vi "Peak_removal_diag.vi"(10 "tolerance (Deviation)":dbl, 11 "Offset removed":cluster{"xi used":dbl[], "yi":dbl[]}(graph)) -> (2 "Tolerance Level":dbl, 3 "XY Graph":cluster{"xi used":dbl[], "yi":dbl[]}(graph))   [LabVIEW 2015]
uses:
  <vilib>/Analysis/NI_AALBase.lvlib
panel:
  out "yi":dbl[](array[numeric])
  out "xi used":dbl[](array[numeric])
  out "XY Graph 2":cluster{"xi used":dbl[], "yi":dbl[]}(graph)
  out "standard deviation":dbl format="%0.2f"
  out "mean":dbl format="%0.2f"
  out "yi 2":dbl[](array[numeric])
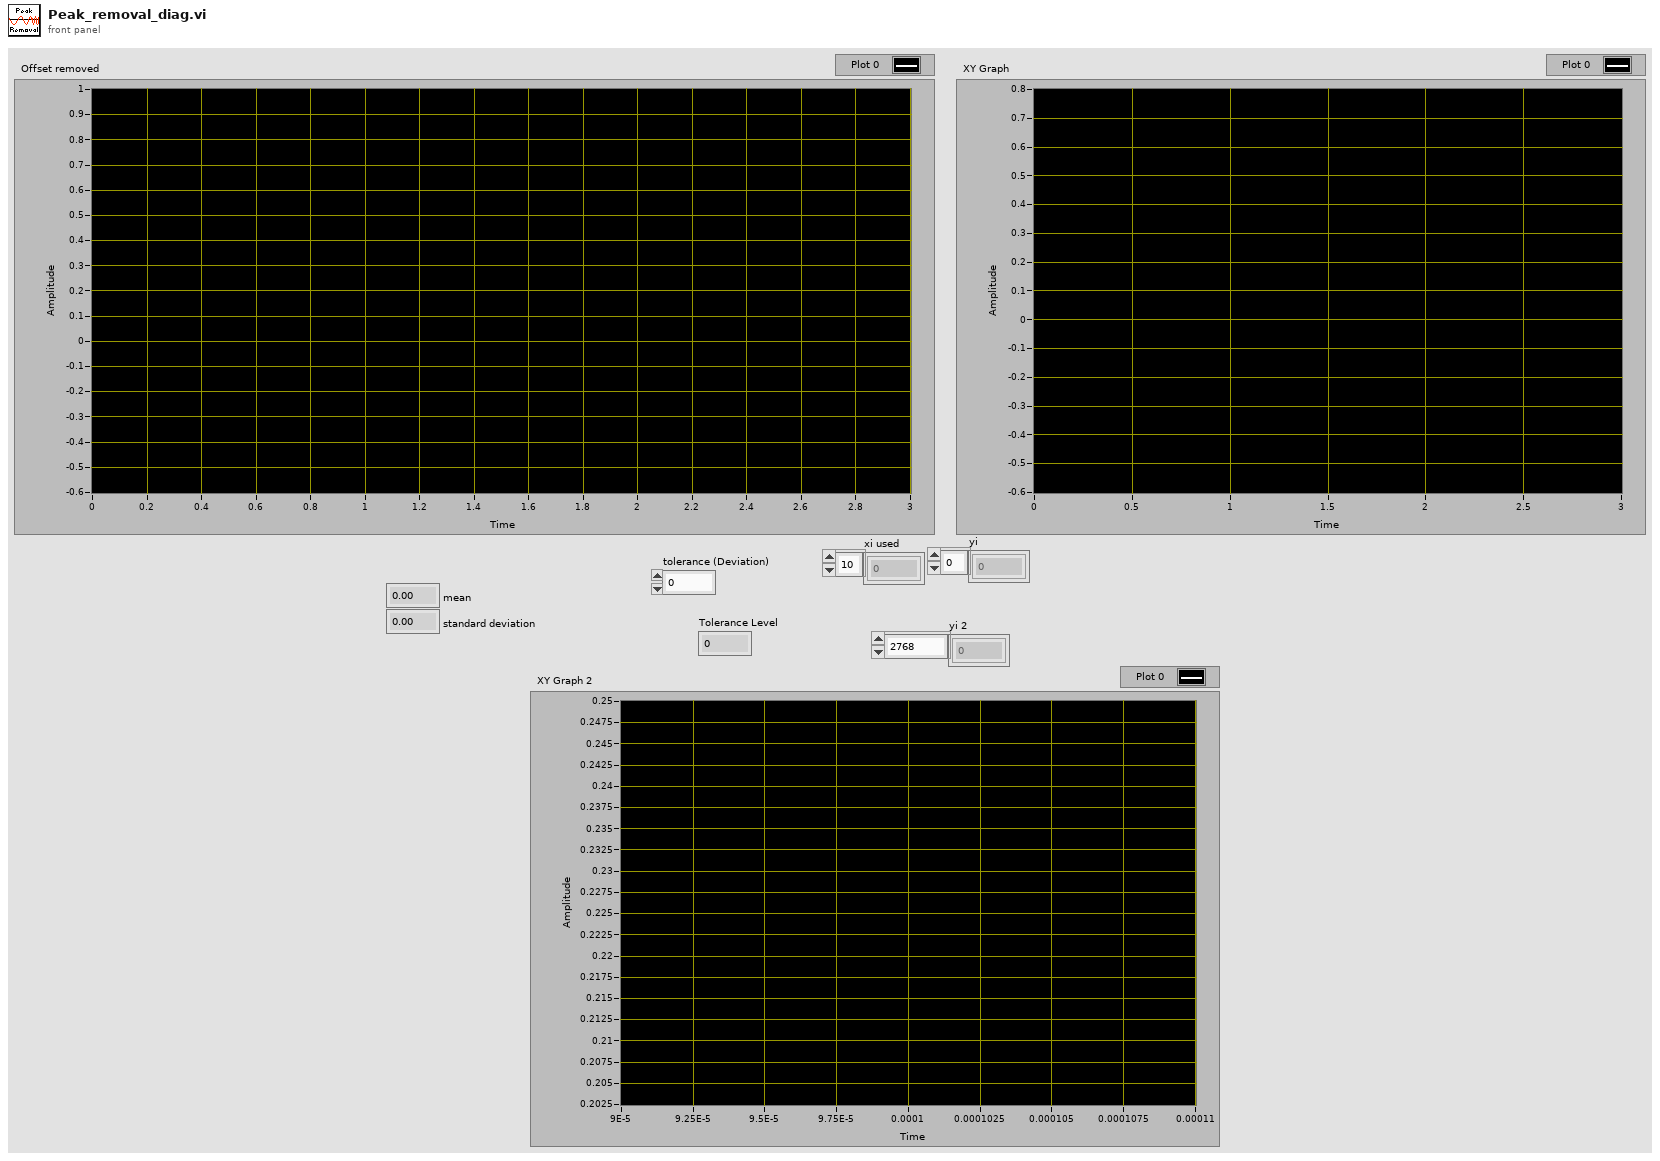
[diagram p1: front panel]
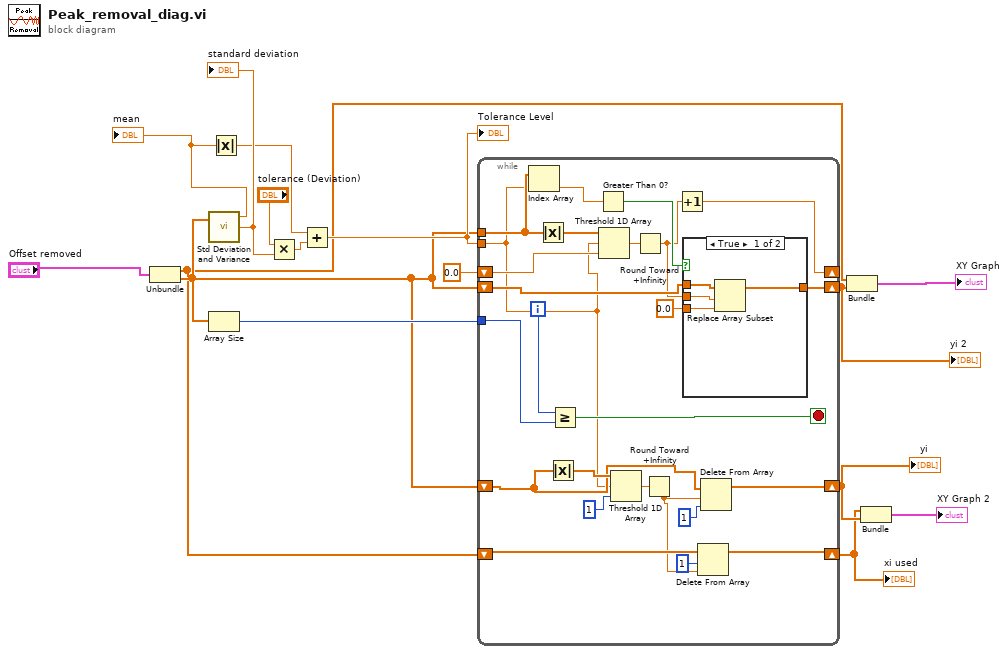
[diagram p0: block diagram]
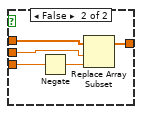
[diagram p2: hidden frame]
diagram:
  n1 = Unbundle("Offset removed") -> ("xi used"=w6:dbl[], "yi"=w7:dbl[])
  n2 = call <vilib>:"Std Deviation and Variance.vi"("X"=w7) -> ("mean"=w2:dbl, "standard deviation"=w16:dbl)  [unwired: 1 in, 1 out]
  "mean" <- w2
  "standard deviation" <- w16
  n3 = Array Size(array=w7) -> (size(s)=w12:i32)
  n4 = Absolute Value(x=w2) -> (abs(x)=w1:dbl)
  n5 = Multiply(x="tolerance (Deviation)", y=w16) -> (x*y=w14:dbl)
  n6 = Add(x=w1, y=w14) -> (x+y=w13:dbl)
  "Tolerance Level" <- w13
  n7 = while {
    tunnel: w7 -> [w34]
    tunnel: w13 -> [w22]
    shift-right: [w38] -> _
    shift-left: 0.0 -> [w33]
    shift-right: [w40] -> w10
    shift-left: w7 -> [w30]
    tunnel: w12 -> [w36]
    shift-right: [w24] -> w5
    shift-left: w7 -> [w25]
    shift-right: [w20] -> w4
    shift-left: w6 -> [w21]
    i -> [w37]
    stop <- w39 stop-if-true
    n8 = Index Array(array=w34, index=w22) -> (element=w32:dbl)
    n9 = Absolute Value(x=w34) -> (abs(x)=w35:dbl[])
    n10 = Absolute Value(x=w25) -> (abs(x)=w27:dbl[])
    n11 = Greater Or Equal?(x=w37, y=w36) -> (x >= y?=w39:bool)
    n12 = Greater Than 0?(x=w32) -> (x > 0?=w31:bool)
    n13 = Threshold 1D Array(1:w33, 2:w22, 3:w35) -> (0:w41:dbl)
    n14 = Threshold 1D Array(1:1 ("start index (0)"), 2:w22, 3:w27) -> (0:w26:dbl)
    n15 = Round Toward +Infinity(x=w41) -> (ceil(x): smallest int >= x=w29:dbl)
    n16 = Round Toward +Infinity(x=w26) -> (ceil(x): smallest int >= x=w18:dbl)
    n17 = Increment(x=w29) -> (x+1=w38:dbl)
    n18 = case shown="True" w31 {
      tunnel: [w45 w50] -> w40
      tunnel: w30 -> [w44 w49]
      tunnel: w29 -> [w43 w48]
      tunnel: 0.0 -> [w42 w46]
      frame True {
        n19 = Replace Array Subset(array=w44, new element=w42, index=w43) -> (w45:dbl[])
      }
      frame False {
        n20 = Negate(x=w46) -> (-x=w47:dbl)
        n21 = Replace Array Subset(array=w49, new element=w47, index=w48) -> (w50:dbl[])
      }
    }
    n22 = Delete From Array(array=w21, length=1, index=w18) -> (array with subset deleted=w20:dbl[])  [unwired: 1 out]
    n23 = Delete From Array(array=w25, length=w18, index=1) -> (array with subset deleted=w24:dbl[])  [unwired: 1 out]
  }
  "yi 2" <- w10
  "xi used" <- w4
  "yi" <- w5
  n24 = Bundle("xi used"=w6, "yi"=w10) -> (→"XY Graph":cluster{"xi used":dbl[], "yi":dbl[]})  [unwired: 1 in]
  n25 = Bundle("xi used"=w4, "yi"=w5) -> (→"XY Graph 2":cluster{"xi used":dbl[], "yi":dbl[]})  [unwired: 1 in]
